vi "Set Value.vi"(8 "Error In":errorcluster, 10 "Value":dbl, 11 "Number Widget In":refnum<class "5. Number Widget.lvclass">) -> (0 "Error Out":errorcluster, 3 "Number Widget Out":refnum<class "5. Number Widget.lvclass">)   [LabVIEW 2014, in "Hello World - Introduction to Widgets.lvlib" / "5. Number Widget.lvclass"]
doc: "Copyright (c) 2016 Sze Howe Koh\nThis code is licensed under the MIT license"
uses:
  5. Number Widget.lvclass
  5. Number Widget.lvclass/5. Number Widget.ctl
  src/LabVIEW/Qwt/QwtAbstractSlider/QwtAbstractSlider.lvclass
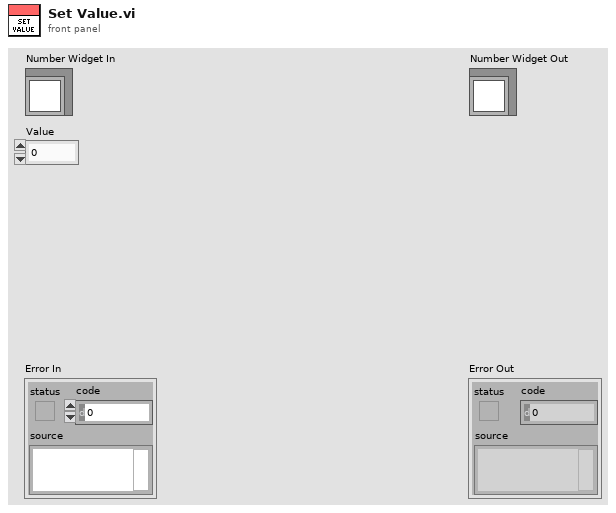
[diagram p1: front panel]
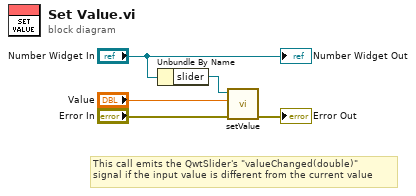
[diagram p0: block diagram]
diagram:
  # "This call emits the QwtSlider's \"valueChanged(double)\"\nsignal if the input value is different from the current value"
  n1 = Unbundle By Name("Number Widget In") -> ("slider"=w3:refnum<class "QwtSlider.lvclass">)
  n2 = call "setValue.vi"("Error In"="Error In", "val"="Value", "QwtAbstractSlider In"=w3) -> ("Error Out"=→"Error Out":errorcluster)  [unwired: 7 in, 1 out]
  "Number Widget Out" <- "Number Widget In"
